vi "Close References To All Libraries And VIs In Project.vi"(8 "error in (no error)":errorcluster, 11 "VI and Library References":T1[](array[typedef])) -> (0 "error out":errorcluster)   [LabVIEW 2020, in "Edit LVProj.lvlib"]
uses:
  <vilib>/Utility/EditLVProj/Edit LVProj.lvlib
  <vilib>/Utility/EditLVProj/Library And VI References.ctl
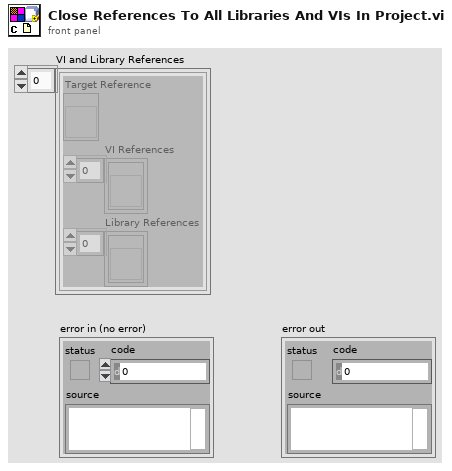
[diagram p1: front panel]
types:
  T1 = typedef "Edit LVProj.lvlib/Library And VI References.ctl" = cluster{"Target Reference":refnum<vi>, "VI References":refnum<vi>[], "Library References":refnum<vi>[]}
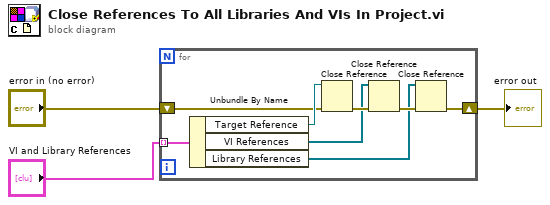
[diagram p0: block diagram]
diagram:
  n1 = for {
    tunnel: "VI and Library References" -> [w11] mode=indexing
    shift-right: [w4] -> w1
    shift-left: "error in (no error)" -> [w5]
    n2 = Unbundle By Name(w11) -> ("Target Reference"=w10:refnum<vi>, "VI References"=w7:refnum<vi>[], "Library References"=w6:refnum<vi>[])
    n3 = Close Reference(reference=w10, error in (no error)=w5) -> (error out=w9:errorcluster)
    n4 = Close Reference(reference=w7, error in (no error)=w9) -> (error out=w8:errorcluster)
    n5 = Close Reference(reference=w6, error in (no error)=w8) -> (error out=w4:errorcluster)
  }
  "error out" <- w1
